vi "PDE_SpMtrx_CG Solver_Check Input.vi"(6 "termination in":cluster{"max iter":i32, "tolerance":dbl}={"max iter"=200, "tolerance"=1e-08}, 8 "error in (no error)":errorcluster, 9 "X0 In":dbl[](array[numeric]), 10 "RHS":dbl[](array[numeric]), 11 "Sparse Mtrx":T1) -> (0 "error out":errorcluster, 2 "termination out":cluster{"max iter":i32, "tolerance":dbl}, 3 "X0 Out":dbl[](array[numeric]))   [LabVIEW 2017, in "NI_PDE.lvlib"]
uses:
  <vilib>/gmath/NI_PDE.lvlib
  <vilib>/gmath/pde.llb/Common/PDE_Sparse Mtrx.ctl
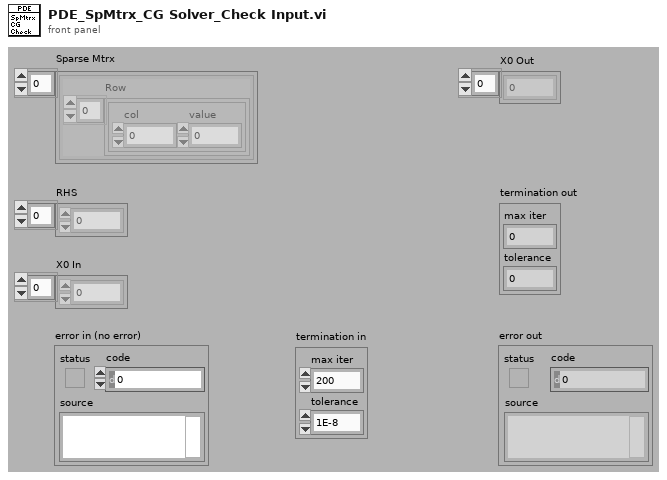
[diagram p1: front panel]
types:
  T1 = typedef "NI_PDE.lvlib/PDE_Sparse Mtrx.ctl" = cluster{"Row":cluster{"col":i32, "value":dbl}[]}[]
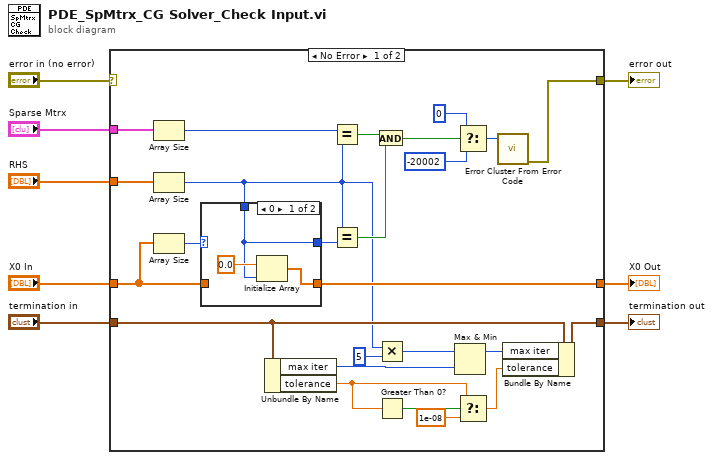
[diagram p0: block diagram]
diagram:
  n1 = case shown="No Error" "error in (no error)" {
    selector: "error in (no error)" -> [_ w41]
    tunnel: "termination in" -> [w23 w40]
    tunnel: "X0 In" -> [w29 w39]
    tunnel: "Sparse Mtrx" -> [w33 _]
    tunnel: "RHS" -> [w32 _]
    tunnel: [w14 w41] -> w3
    tunnel: [w27 w39] -> w2
    tunnel: [w21 w40] -> w1
    frame No Error {
      n2 = Array Size(array=w33) -> (size(s)=w31:i32)
      n3 = Array Size(array=w32) -> (size(s)=w11:i32)
      n4 = Array Size(array=w29) -> (size(s)=w30:i32)
      n5 = case shown="0" w30 {
        selector: w30 -> [_ w37]
        tunnel: [w36 w38] -> w27
        tunnel: w29 -> [_ w38]
        tunnel: w11 -> [w34 _]
        tunnel: [w34 w37] -> w28
        frame 0 {
          n6 = Initialize Array(0.0 ("element"), w34) -> (w36:dbl[])
        }
        frame 1, Default {
        }
      }
      n7 = Unbundle By Name(w23) -> ("max iter"=w12:i32, "tolerance"=w24:dbl)
      n8 = Equal?(x=w31, y=w11) -> (x = y?=w20:bool)
      n9 = Equal?(x=w11, y=w28) -> (x = y?=w19:bool)
      n10 = And(x=w20, y=w19) -> (x .and. y?=w18:bool)
      n11 = Multiply(x=w11, y=5) -> (x*y=w10:i32)
      n12 = Greater Than 0?(x=w24) -> (x > 0?=w25:bool)
      n13 = Max & Min(x=w10, y=w12) -> (max(x,y)=w13:i32)  [unwired: 1 out]
      n14 = Select(t=0, s=w18, f=-20002) -> (s? t:f=w15:i32)
      n15 = Select(t=w24, s=w25, f=1e-08) -> (s? t:f=w22:dbl)
      n16 = call <vilib>:"Error Cluster From Error Code.vi"("error code (0)"=w15) -> ("error out"=w14:errorcluster)  [unwired: 2 in, 6 out]
      n17 = Bundle By Name(cluster=w23, "max iter"=w13, "tolerance"=w22) -> (w21:cluster{"max iter":i32, "tolerance":dbl})
    }
    frame Error {
    }
  }
  "X0 Out" <- w2
  "error out" <- w3
  "termination out" <- w1
